vi "Initialize.vi"(8 "error in (no error)":errorcluster, 10 "config path":path, 11 "LightBox in":refnum<class "LightBox.lvclass">) -> (0 "error out":errorcluster, 3 "LightBox out":refnum<class "LightBox.lvclass">)   [LabVIEW 2016, in "LightBox.lvclass"]
uses:
  LightBox.lvclass
  Lamp.lvclass
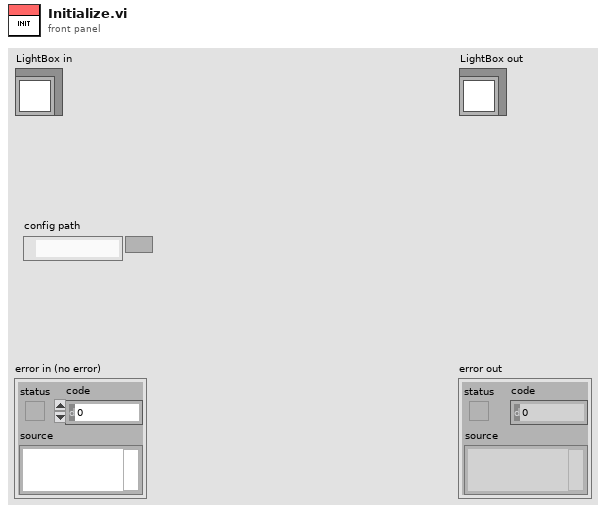
[diagram p1: front panel]
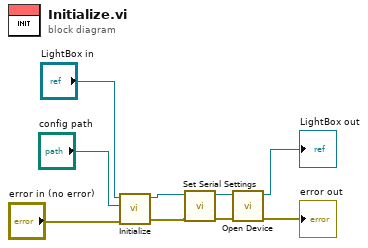
[diagram p0: block diagram]
diagram:
  n1 = call-parent "Initialize.vi"("error in (no error)"="error in (no error)", "config path"="config path", "Lamp in"="LightBox in") -> ("error out"=w5:errorcluster, "Lamp out"=w6:refnum<class "LightBox.lvclass">)  [unwired: 7 in]
  n2 = call-dynamic "Set Serial Settings.vi"("error in (no error)"=w5, "LightBox in"=w6) -> ("error out"=w3:errorcluster, "LightBox out"=w4:refnum<class "LightBox.lvclass">)  [unwired: 8 in]
  n3 = call-dynamic "Open Device.vi"("error in (no error)"=w3, "LightBox in"=w4) -> ("error out"=→"error out":errorcluster, "LightBox out"=→"LightBox out":refnum<class "LightBox.lvclass">)  [unwired: 8 in]
